vi "testGetServerNotifier(base).vi"(8 "error in (no error)":errorcluster) -> (0 "error out":errorcluster)   [LabVIEW 2018]
doc: "Test the getServerNotifier.vi."
uses:
  src/TcpServer/TcpServer.lvclass
  src/TcpServer/TcpServer.lvclass/TcpServer.ctl
  src/TcpServerBase/TcpServerBase.lvclass/TcpServerBase.ctl
  src/TcpServerCmd/TcpServerCmd.lvclass
  home/pcortes/Documents/github/ts_labview_tcp_json/src/TcpServerBase/TcpServerBase.lvclass
  <vilib>/addons/_JKI Toolkits/Caraya/classes/Assert/Assert Equal Type_Variant.vi
  <vilib>/addons/_JKI Toolkits/Caraya/classes/Test/Test.lvclass
  <vilib>/addons/_JKI Toolkits/Caraya/classes/Assert/Assert.lvclass
  src/TcpServerBase/TcpServerBase.lvclass
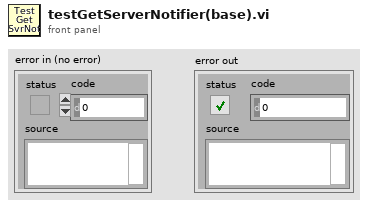
[diagram p1: front panel]
types:
  T1 = cluster{"connectionStatus":bool, "errorSource":string}
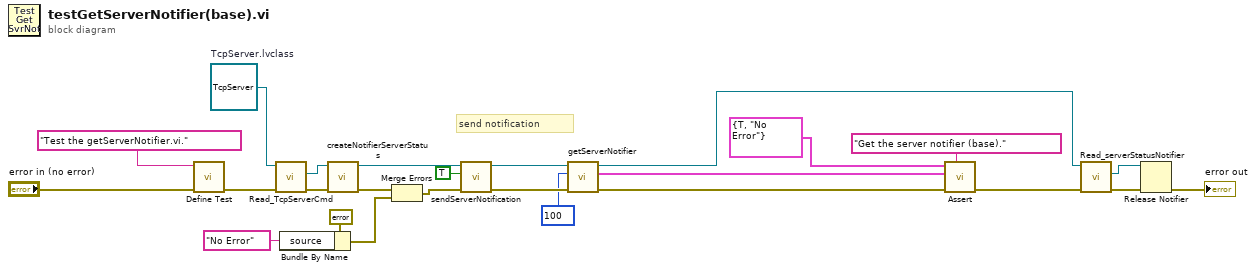
[diagram p0: block diagram]
diagram:
  w13 = refnum<class "TcpServer.lvclass"> refnum  # TcpServer.lvclass
  # "send notification"
  n1 = call <vilib>:"Define Test.vi"("error in (no error)"="error in (no error)", "Label (VI Title)"="Test the getServerNotifier.vi.") -> ("error out"=w10:errorcluster)  [unwired: 9 in]
  n2 = call "Read_TcpServerCmd.vi"("error in (no error)"=w10, "TcpServer in"=w13) -> ("error out"=w11:errorcluster, "TcpServerCmd.lvclass"=w12:refnum<class "TcpServerCmd.lvclass">)  [unwired: 7 in, 1 out]
  n3 = Bundle By Name(cluster=errorcluster {"status"=FALSE, "code"=0, "source"=""} ("error in (no error)"), "source"="No Error") -> (w16:errorcluster)
  n4 = call "createNotifierServerStatus.vi"("error in (no error)"=w11, "tcpServerBase in"=w12) -> ("error out"=w15:errorcluster, "tcpServerBase out"=w22:refnum<class "TcpServerCmd.lvclass">)  [unwired: 8 in]
  n5 = Merge Errors(w15, w16) -> (w17:errorcluster)
  n6 = call "sendServerNotification.vi"("error in (no error)"=w17, "connectionStatus"=TRUE ("serverStatus"), "TcpServerBase in"=w22) -> ("error out"=w8:errorcluster, "TcpServerBase out"=w9:refnum<class "TcpServerCmd.lvclass">)  [unwired: 7 in]
  n7 = call "getServerNotifier.vi"("error in (no error)"=w8, "notifier timeout"=100 ("Timeout Notifier"), "TcpServerBase in"=w9) -> ("error out"=w5:errorcluster, "connStatusCluster"=w6:T1, "TcpServerBase out"=w2:refnum<class "TcpServerCmd.lvclass">)  [unwired: 5 in, 1 out]
  n8 = call-poly <vilib>:"Assert.vi"("Label"="Get the server notifier (base).", "error in (no error)"=w5, "Y"=w6, "X"=T1 {"connectionStatus"=TRUE, "errorSource"="No Error"} ("notification")) -> ("error out"=w14:errorcluster)  [unwired: 7 in]
  n9 = call "Read_serverStatusNotifier.vi"("error in (no error)"=w14, "TcpServerBase in"=w2) -> ("error out"=w4:errorcluster, "serverStatusNotifier"=w1:refnum<notifier>)  [unwired: 7 in, 1 out]
  n10 = Release Notifier(notifier=w1, error in (no error)=w4) -> (error out=→"error out":errorcluster)  [unwired: 1 in, 2 out]
